vi "Activate-selected-motors.vi"(8 "error in (no error)":errorcluster, 10 "Selected motors":T1, 11 "Available motors in":refnum<class "Motor-assembly.lvclass">) -> (0 "error out":errorcluster, 3 "Available motors out":refnum<class "Motor-assembly.lvclass">)   [LabVIEW 2013, in "PowderDeposition.lvlib" / "Motor-assembly.lvclass"]
doc: "Activate the motors that are selected - correspondig button pressed - but not yet active."
uses:
  Motor-assembly.lvclass
  Motor-selection.ctl
  Motor/Motor.lvclass
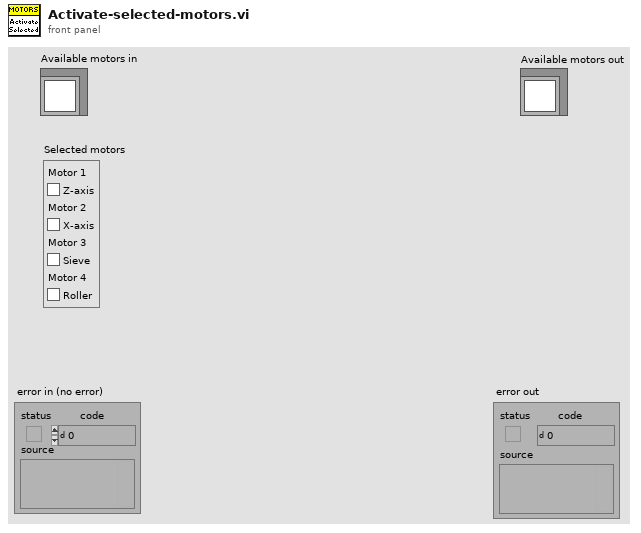
[diagram p1: front panel]
types:
  T1 = typedef "PowderDeposition.lvlib/Motor-assembly.lvclass/Motor-selection.ctl" = cluster{"Motor 1":bool, "Motor 2":bool, "Motor 3":bool, "Motor 4":bool}
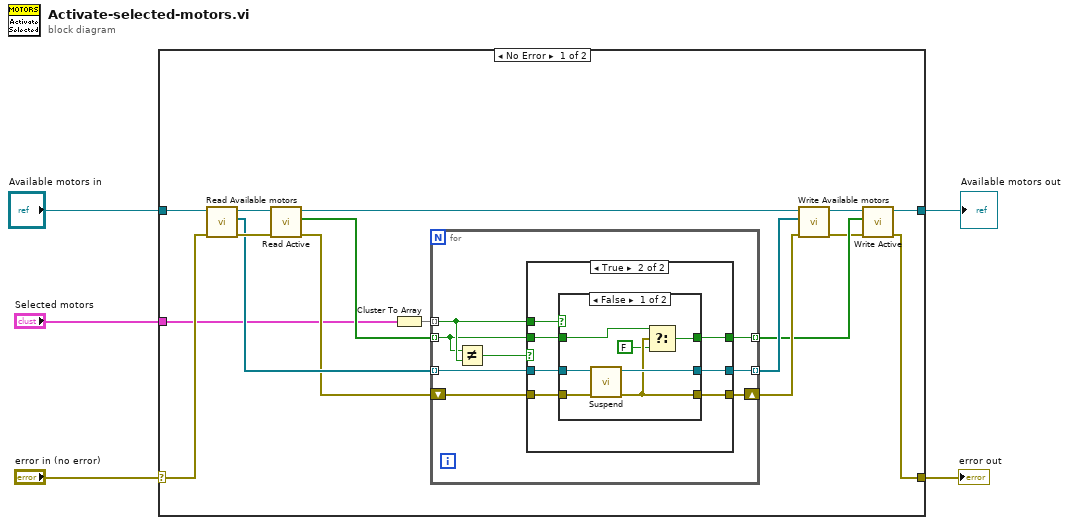
[diagram p0: block diagram]
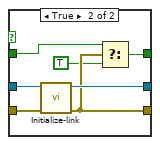
[diagram p3: hidden frame]
diagram:
  n1 = case shown="No Error" "error in (no error)" {
    selector: "error in (no error)" -> [w10 w56]
    tunnel: [w7 w56] -> w4
    tunnel: "Available motors in" -> [w9 w55]
    tunnel: [w8 w55] -> w2
    tunnel: "Selected motors" -> [w6 _]
    frame No Error {
      n2 = call-dynamic "Read Available motors.vi"("error in (no error)"=w10, "Available motors in"=w9) -> ("error out"=w21:errorcluster, "Available motors"=w18:refnum<class "Motor.lvclass">[], "Available motors out"=w22:refnum<class "Motor-assembly.lvclass">)  [unwired: 7 in]
      n3 = call-dynamic "Read Active.vi"("error in (no error)"=w21, "Available motors in"=w22) -> ("error out"=w17:errorcluster, "Active?"=w19:bool[], "Available motors out"=w14:refnum<class "Motor-assembly.lvclass">)  [unwired: 7 in]
      n4 = Cluster To Array(cluster=w6) -> (array=w20:bool[])
      n5 = for {
        tunnel: w20 -> [w24] mode=indexing
        tunnel: w19 -> [w23] mode=indexing
        tunnel: w18 -> [w30] mode=indexing
        tunnel: [w29] -> w15 mode=indexing
        shift-right: [w27] -> w16
        shift-left: w17 -> [w28]
        tunnel: [w26] -> w13 mode=indexing
        n6 = Not Equal?(x=w23, y=w24) -> (x != y?=w25:bool)
        n7 = case shown="True" w25 {
          tunnel: w24 -> [_ w40]
          tunnel: w30 -> [w32 w39]
          tunnel: [w32 w38] -> w29
          tunnel: w28 -> [w31 w37]
          tunnel: [w31 w36] -> w27
          tunnel: [w33 w35] -> w26
          tunnel: w23 -> [w33 w34]
          frame False {
          }
          frame True {
            n8 = case shown="False" w40 {
              tunnel: w39 -> [w47 w54]
              tunnel: [w45 w53] -> w38
              tunnel: w37 -> [w46 w52]
              tunnel: [w42 w50] -> w36
              tunnel: [w44 w51] -> w35
              tunnel: w34 -> [w43 w49]
              frame False {
                n9 = call-dynamic "Suspend.vi"("error in (no error)"=w46, "Motor in"=w47) -> ("error out"=w42:errorcluster, "Motor out"=w45:refnum<class "Motor.lvclass">)  [unwired: 8 in]
                n10 = Select(t=w43, s=w42, f=FALSE) -> (s? t:f=w44:bool)
              }
              frame True {
                n11 = call-dynamic "Initialize-link.vi"("error in (no error)"=w52, "Motor in"=w54) -> ("error out"=w50:errorcluster, "Motor out"=w53:refnum<class "Motor.lvclass">)  [unwired: 8 in]
                n12 = Select(t=w49, s=w50, f=TRUE) -> (s? t:f=w51:bool)
              }
            }
          }
        }
      }
      n13 = call-dynamic "Write Available motors.vi"("error in (no error)"=w16, "Available motors"=w15, "Available motors in"=w14) -> ("error out"=w11:errorcluster, "Available motors out"=w12:refnum<class "Motor-assembly.lvclass">)  [unwired: 7 in]
      n14 = call-dynamic "Write Active.vi"("error in (no error)"=w11, "Active?"=w13, "Available motors in"=w12) -> ("error out"=w7:errorcluster, "Available motors out"=w8:refnum<class "Motor-assembly.lvclass">)  [unwired: 7 in]
    }
    frame Error {
    }
  }
  "error out" <- w4
  "Available motors out" <- w2
